vi "BRig_dataBlock_c_T2R_R.vi"() -> (2 "output_c_T2R_R":i32)   [LabVIEW 2014]
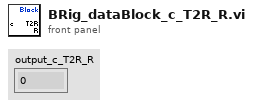
[diagram p1: front panel]
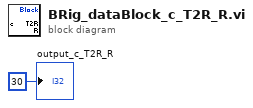
[diagram p0: block diagram]
diagram:
  "output_c_T2R_R" <- 30 ("output_iBlock")
